vi "Load App.vi"(8 "error in (no error)":errorcluster, 11 "Status Notifier":refnum<notifier>) -> (0 "error out":errorcluster)   [LabVIEW 2018, in "MWWL Verification.lvlib" / "MWWL Verification.lvclass"]
doc: "Load the application into memory and start it running. The input notifier is used to send text to the splash screen to tell the user what stage the load process is in."
uses:
  MWWL Verification.lvclass
  C:/Program Files (x86)/National Instruments/LabVIEW 2018/vi.lib/ActorFramework/Actor/Actor.lvclass
  <vilib>/ActorFramework/Actor/Actor.lvclass
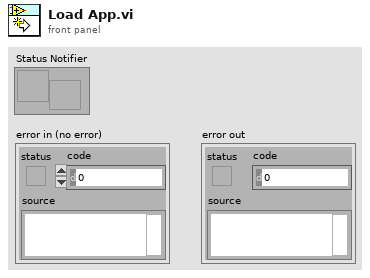
[diagram p1: front panel]
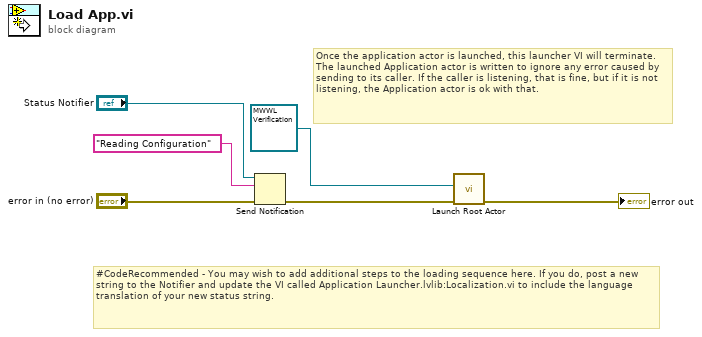
[diagram p0: block diagram]
diagram:
  # "Once the application actor is launched, this launcher VI will terminate. The launched Application actor is written to ignore any error caused by sending to its caller. If the caller is listening, that is fine, but if it is not listening, the Application actor is ok with that."
  # "#CodeRecommended - You may wish to add additional steps to the loading sequence here. If you do, post a new string to the Notifier and update the VI called Application Launcher.lvlib:Localization.vi to include the language translation of your new status string."
  n1 = Send Notification(notification="Reading Configuration", notifier="Status Notifier", error in (no error)="error in (no error)") -> (error out=w2:errorcluster)  [unwired: 1 out]
  n2 = call <vilib>:"Launch Root Actor.vi"("error in (no error)"=w2, "Actor"=refnum<class "MWWL Verification.lvclass"> refnum ("MWWL Verification.lvlib:MWWL Verification.lvclass")) -> ("error out"=→"error out":errorcluster)  [unwired: 8 in, 1 out]
